vi "Get UI Details.vi"() -> ()   [LabVIEW 2021, in "Waveform Mode_Channel Ganging.lvlib"]
uses:
  Waveform Mode_Channel Ganging.lvlib
  <vilib>/Plug-In SDKs/Measurements/Helpers/TypeDefs/User Interface Information.ctl
  <vilib>/Plug-In SDKs/Measurements/NI Measurement Plug-In SDK.lvlib
panel:
  out "error out":errorcluster
  in  "error in":errorcluster
  out "user interface details":T1[](array[typedef])
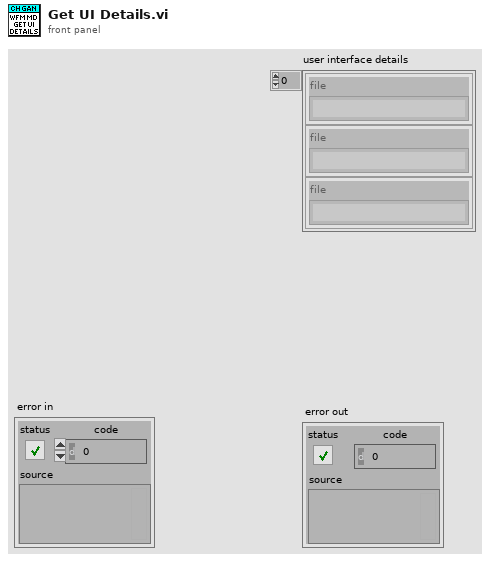
[diagram p1: front panel]
types:
  T1 = typedef "NI Measurement Plug-In SDK.lvlib/User Interface Information.ctl" = cluster{"file":string}
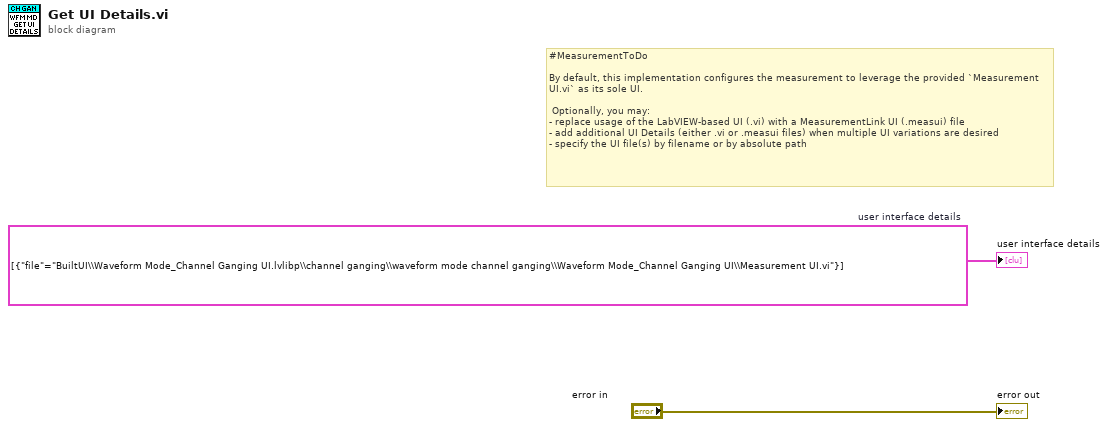
[diagram p0: block diagram]
diagram:
  w2 = T1[] [{"file"="BuiltUI\\Waveform Mode_Channel Ganging UI.lvlibp\\channel ganging\\waveform mode channel ganging\\Waveform Mode_Channel Ganging UI\\Measurement UI.vi"}]  # user interface details
  # "#MeasurementToDo\n\nBy default, this implementation configures the measurement to leverage the provided `Measurement UI.vi` as its sole UI.\n\n Optionally, you may:\n- replace usage of the LabVIEW-based UI (.vi) with a MeasurementLink UI (.measui) file\n- add additional UI Details (either .vi or .measui files) when multiple UI variations are desired\n- specify the UI file(s) by filename or by absolute path"
  "user interface details" <- w2
  "error out" <- "error in"
